vi "Get Variable List.vi"(8 "Error In":errorcluster, 9 "Selected Libraries":i32[](listbox), 10 "library URL":string[](array[string]), 11 "library Name":string[](array[string])) -> (0 "Error Out":errorcluster, 1 "Selected Library Names":string[](array[string]), 2 "Selected Library URLs":string[](array[string]), 3 "Variable":T1)   [LabVIEW 2014]
doc: "<B>Copyright</B>: (c) MHWirth 2015. All rights reserved.\n\nThis subVI provides a list of variable information (name + URLs) for the selected deployed process/processes (library/libraries)."
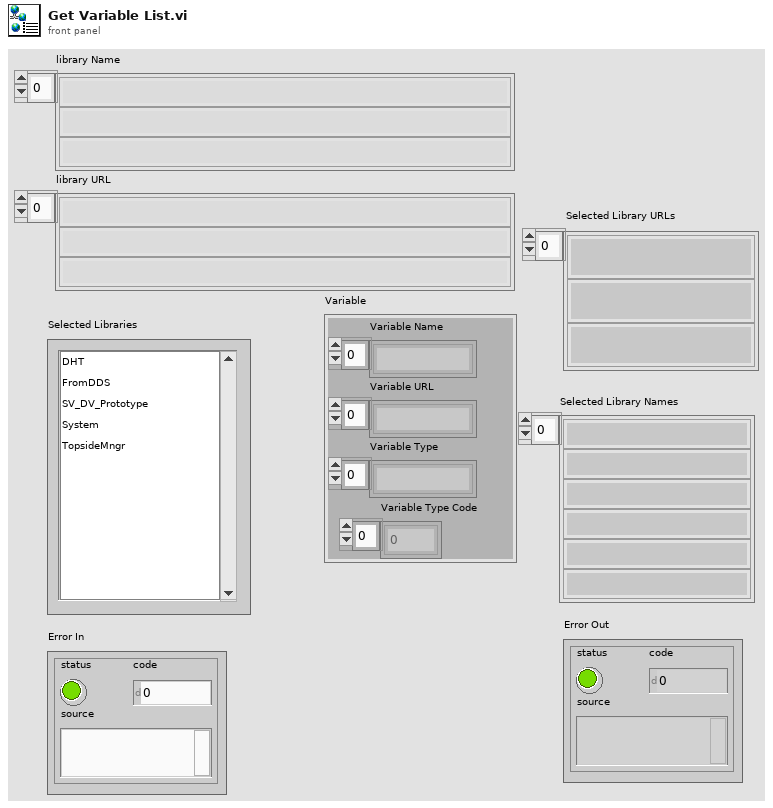
[diagram p1: front panel]
types:
  T1 = cluster{"Variable Name":string[], "Variable URL":string[], "Variable Type":string[], "Variable Type Code":i32[]}
  T2 = cluster{"Number of Variables":i32, "Variable/Parent Name array":string[][], "URL array":string[], "Type array":string[]}
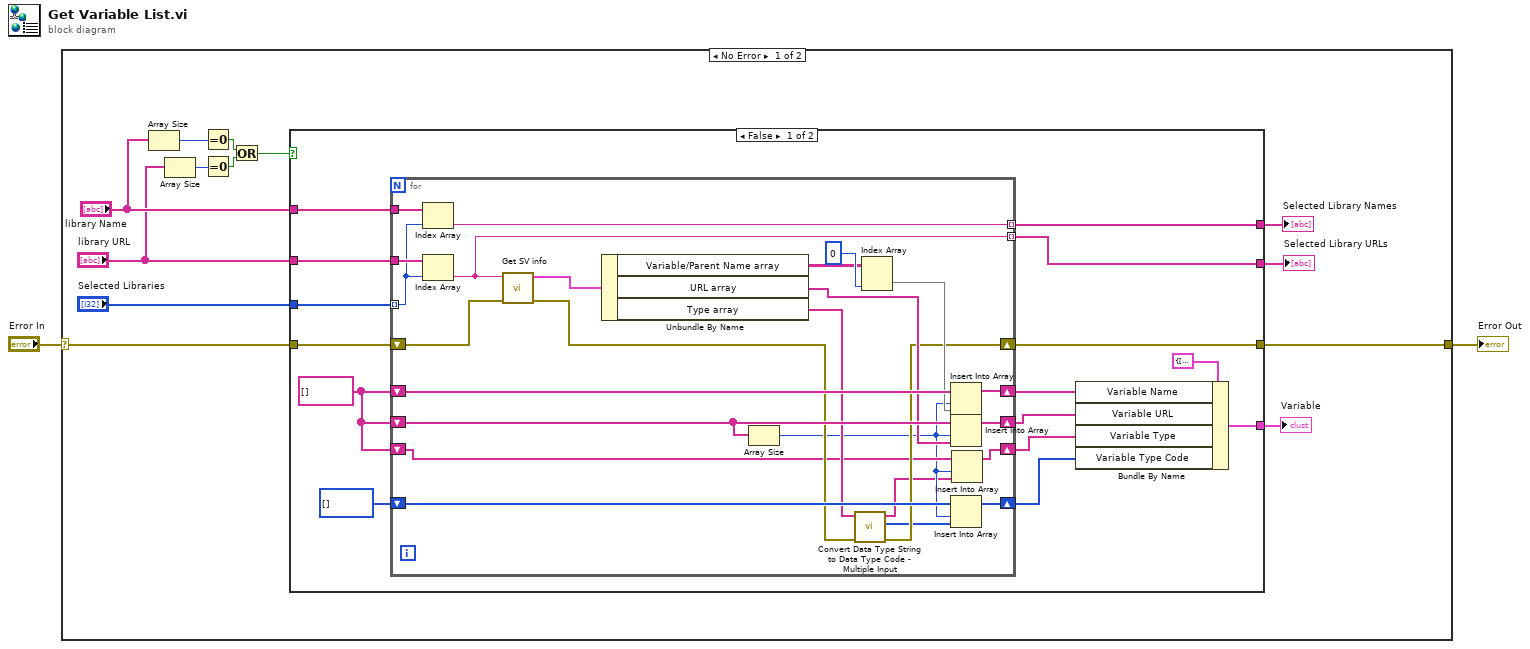
[diagram p0: block diagram]
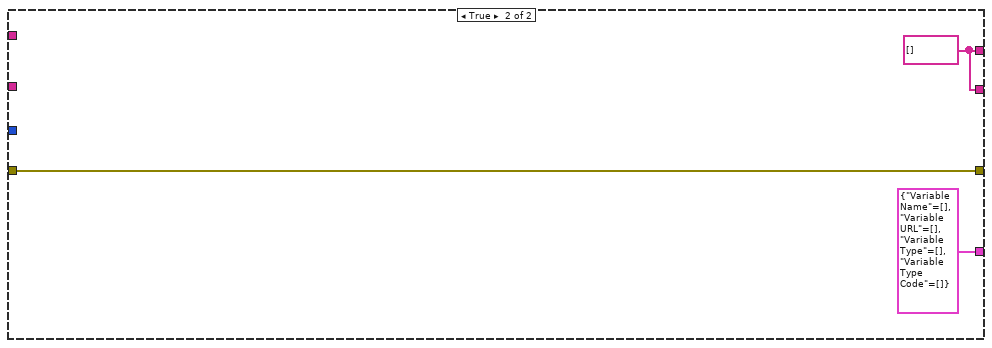
[diagram p2: hidden frame]
diagram:
  n1 = case shown="No Error" "Error In" {
    selector: "Error In" -> [w14 w59]
    tunnel: [w13 w59] -> w1
    frame No Error {
      n2 = Array Size(array="library Name") -> (size(s)=w7:i32)
      n3 = Array Size(array="library URL") -> (size(s)=w6:i32)
      n4 = Equal To 0?(x=w7) -> (x = 0?=w4:bool)
      n5 = Equal To 0?(x=w6) -> (x = 0?=w5:bool)
      n6 = Or(x=w4, y=w5) -> (x .or. y?=w3:bool)
      n7 = case shown="False" w3 {
        tunnel: "Selected Libraries" -> [w30 _]
        tunnel: "library URL" -> [w29 _]
        tunnel: w14 -> [w28 w57]
        tunnel: [w25 w57] -> w13
        tunnel: [w24 w58] -> w12
        tunnel: [w23 w58] -> w11
        tunnel: [w17 T1 {"Variable Name"=[], "Variable URL"=[], "Variable Type"=[], "Variable Type Code"=[]} ("output cluster")] -> w10
        tunnel: "library Name" -> [w16 _]
        frame False {
          w21 = string[] []
          n8 = for {
            tunnel: w30 -> [w50] mode=indexing
            tunnel: w29 -> [w55]
            shift-right: [w37] -> w25
            shift-left: w28 -> [w47]
            shift-right: [w53] -> w27
            shift-left: w21 -> [w54]
            shift-right: [w35] -> w26
            shift-left: w21 -> [w52]
            tunnel: w16 -> [w51]
            tunnel: [w49] -> w24 mode=indexing
            tunnel: [w48] -> w23 mode=indexing
            shift-right: [w42] -> w19
            shift-left: i32[] [] -> [w41]
            shift-right: [w31] -> w18
            shift-left: w21 -> [w34]
            n9 = Index Array(array=w51, index=w50) -> (element=w49:string)
            n10 = Index Array(array=w55, index=w50) -> (element=w48:string)
            n11 = call "Get SV info.vi"("Error In"=w47, "container refnum in"=w48) -> ("Error Out"=w38:errorcluster, "Deployed Shared Variable Information"=w46:T2)  [unwired: 7 in, 1 out]
            n12 = Unbundle By Name(w46) -> ("Variable/Parent Name array"=w44:string[][], "URL array"=w40:string[], "Type array"=w39:string[])
            n13 = Array Size(array=w52) -> (size(s)=w33:i32)
            n14 = call "Convert Data Type String to Data Type Code - Multiple Input.vi"("Error In"=w38, "Type Array"=w39) -> ("Error Out"=w37:errorcluster, "Type code Array"=w36:i32[], "Type Array"=w32:string[])  [unwired: 7 in]
            n15 = Index Array(array=w44, index (col)=0 ("disabled index (col)")) -> (element=w43:string[])  [unwired: 1 in]
            n16 = Insert Into Array(array=w54, index=w33, new element=w43) -> (w53:string[])
            n17 = Insert Into Array(array=w52, index=w33, new element=w40) -> (w35:string[])
            n18 = Insert Into Array(array=w41, index=w33, new element=w36) -> (w42:i32[])
            n19 = Insert Into Array(array=w34, index=w33, new element=w32) -> (w31:string[])
          }
          n20 = Bundle By Name(cluster=T1 {"Variable Name"=[], "Variable URL"=[], "Variable Type"=[], "Variable Type Code"=[]} ("output cluster"), "Variable Name"=w27, "Variable URL"=w26, "Variable Type"=w18, "Variable Type Code"=w19) -> (w17:T1)
        }
        frame True {
          w58 = string[] []
        }
      }
      "Selected Library Names" <- w12
      "Selected Library URLs" <- w11
      "Variable" <- w10
    }
    frame Error {
    }
  }
  "Error Out" <- w1
